vi "Sliding Average.vi"(9 "Ln2 Filter Size":i16=10, 11 "Array In":T1=[0.0, 0.0, 0.0, 0.0, 0.0, 0.0, 0.0, 0.0, 0.0, 0.0, 0.0, 0.0, 0.0, 0.0, 0.0, 0.0, 0.0, 0.0, 0.0, 0.0, 0.0, 0.0, 0.0, 0.0, 0.0, 0.0, 0.0, 0.0, 0.0, 0.0, 0.0, 0.0, 0.0, 0.0, 0.0, 0.0, 0.0, 0.0, 0.0, 0.0, 0.0, 0.0, 0.0, 0.0, 0.0, 0.0, 0.0, 0.0, 0.0, 0.0, 0.0, 0.0, 0.0, 0.0] format="%_6g") -> (3 "Filtered Array Out":T1 format="%_6g")   [LabVIEW 2020]
doc: "Author: Scott Hannahs <sth@magnet.fsu.edu>\nCopyright 2018 Florida State University, All rights reserved."
uses:
  SCH Data Controls/SCH Data 2 RT Array.ctl
  SCH Data Controls/SCH Data 2 RT.ctl
  SCH Data Controls/SCH Data Average Sum.ctl
  <vilib>/rvi/Memory/Memory_Emulation/nirvimemoryFastEmulation.vi
  <vilib>/rvi/Memory/Memory_Emulation/nirvimemoryEmulation.vi
  <vilib>/rvi/Emulation/niFpgaEmulationIsFPGAContextNoSignature.vi
  <vilib>/rvi/DataTransferAndStorage/Container/Common/niFpgaContainerGetUniqueNameForEmu.vi
  <vilib>/rvi/Emulation/niFpgaProcessEmulError.vi
  <vilib>/rvi/Emulation/niFpgaSctlEmulationGetInTimedLoop.vi
  <vilib>/rvi/errors/nirviReportUnexpectedCaseInternalError (U32).vi
  <vilib>/rvi/DataTransferAndStorage/Container/XNode/niFpgaContainer.xnode
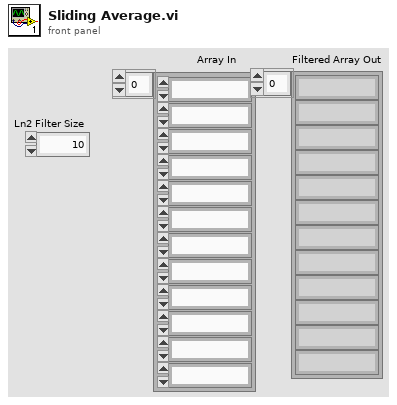
[diagram p1: front panel]
types:
  T1 = typedef "SCH Data 2 RT Array.ctl" = T2[]
  T2 = typedef "SCH Data 2 RT.ctl" = fxp<+/-,38,12>
  T3 = typedef "SCH Data Average Sum.ctl" = fxp<+/-,48,22>
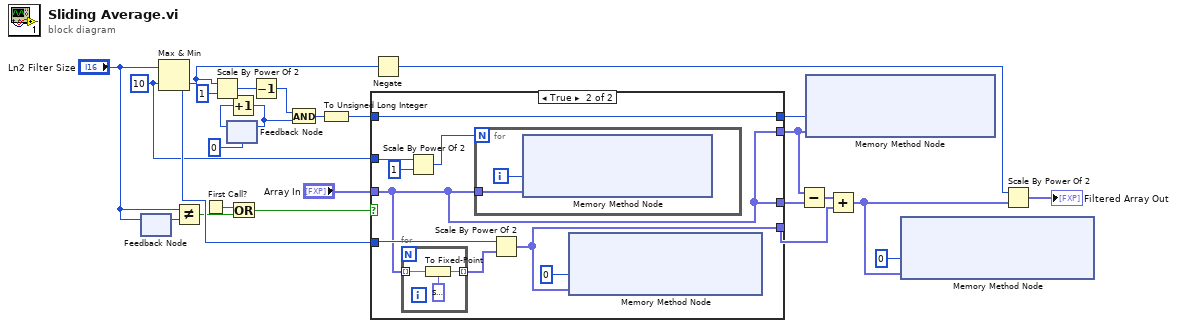
[diagram p0: block diagram]
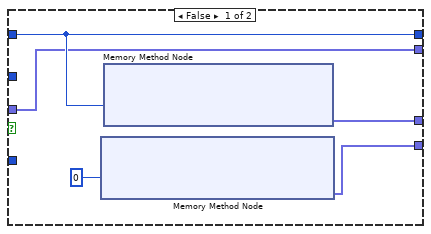
[diagram p2: hidden frame]
diagram:
  w19 = i16 10 ("y")
  n1 = feedback-in #1("Ln2 Filter Size") -> ()
  n2 = feedback #1() -> (w5:i16)  [unwired: 1 in]
  n3 = Max & Min(x="Ln2 Filter Size", y=w19) -> (min(x,y)=w22:i16)  [unwired: 1 out]
  n4 = Not Equal?(x="Ln2 Filter Size", y=w5) -> (x != y?=w6:bool)
  n5 = First Call?() -> (First Call?: T/F=w21:bool)
  n6 = Scale By Power Of 2(n=w22, x=i16 1 ("n")) -> (x*2^n=w23:i16)
  n7 = feedback #2(u16 0 ("y")) -> (w3:u16)
  n8 = Increment(x=w3) -> (x+1=w1:u16)
  n9 = feedback-in #2(w1) -> ()
  n10 = Or(x=w21, y=w6) -> (x .or. y?=w7:bool)
  n11 = Decrement(x=w23) -> (x-1=w11:i16)
  n12 = And(x=w11, y=w1) -> (x .and. y?=w25:u16)
  n13 = To Unsigned Long Integer(number=w25) -> (unsigned 32bit integer=w20:u32)
  n14 = case shown="True" w7 {
    tunnel: w20 -> [w28 w36]
    tunnel: w19 -> [_ w39]
    tunnel: [w28 w36] -> w18
    tunnel: [w30 w31] -> w15
    tunnel: [w29 w32] -> w14
    tunnel: "Array In" -> [w26 w32]
    tunnel: [w26 w32] -> w8
    tunnel: w22 -> [_ w33]
    frame False {
      n15 = xnode ("Memory Method Node")("Address"=u32 0) -> ("Data"=w30:fxp<+/-,48,22>[])  [unwired: 1 in, 1 out]
      n16 = xnode ("Memory Method Node")("Address"=w28) -> ("Data"=w29:fxp<+/-,38,12>[])  [unwired: 1 in, 1 out]
    }
    frame True {
      n17 = for {
        tunnel: [w42] -> w34 mode=indexing
        tunnel: w32 -> [w40] mode=indexing
        n18 = To Fixed-Point(fixed-point type=T3 0.0 ("Numeric"), number=w40) -> (fixed-point=w42:T3)
      }
      n19 = Scale By Power Of 2(n=w39, x=i16 1 ("n")) -> (x*2^n=w37:i16)
      n20 = for {
        N: w37 -> [_]
        tunnel: w32 -> [w43]
        i -> [w44]
        n21 = xnode ("Memory Method Node")("Address"=w44, "Data"=w43) -> ()  [unwired: 1 in, 1 out]
      }
      n22 = Scale By Power Of 2(n=w33, x=w34) -> (x*2^n=w31:T3[])
      n23 = xnode ("Memory Method Node")("Address"=u32 0, "Data"=w31) -> ()  [unwired: 1 in, 1 out]
    }
  }
  n24 = Negate(x=w22) -> (-x=w10:i16)
  n25 = Subtract(x=w8, y=w14) -> (x-y=w16:fxp<+/-,39,13>[])
  n26 = xnode ("Memory Method Node")("Address"=w18, "Data"=w8) -> ()  [unwired: 1 in, 1 out]
  n27 = Add(x=w16, y=w15) -> (x+y=w17:T3[])
  n28 = xnode ("Memory Method Node")("Address"=u32 0, "Data"=w17) -> ()  [unwired: 1 in, 1 out]
  n29 = Scale By Power Of 2(n=w10, x=w17) -> (x*2^n=→"Filtered Array Out":T3[])
